vi "dfd_Validate Subband Counts.vi"(8 "error in (no error)":errorcluster, 10 "band counts":i32) -> (0 "error out":errorcluster, 2 "dup band counts":i32)   [LabVIEW 2017, in "NI_DigFilter_FilterBank.lvlib"]
uses:
  <vilib>/addons/Digital Filter Design/NI_DigFilter_FilterBank.lvlib
  <vilib>/addons/Digital Filter Design/_Misc.llb/dfd_Error Handlers (Single).vi
  <vilib>/addons/Digital Filter Design/NI_DigFilterLicensed.lvlib
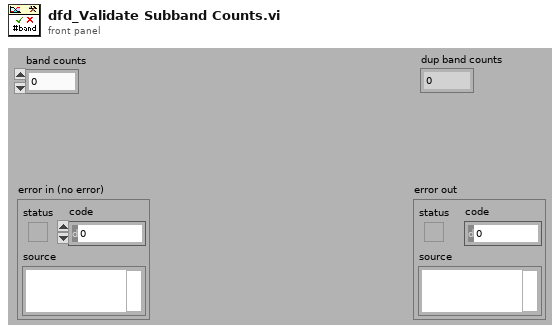
[diagram p1: front panel]
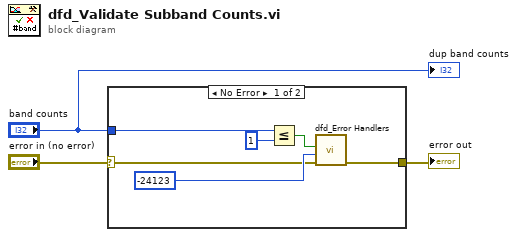
[diagram p0: block diagram]
diagram:
  n1 = case shown="No Error" "error in (no error)" {
    selector: "error in (no error)" -> [w4 w10]
    tunnel: "band counts" -> [w7 _]
    tunnel: [w5 w10] -> w3
    frame No Error {
      n2 = Less Or Equal?(x=w7, y=1) -> (x <= y?=w6:bool)
      n3 = call-poly <vilib>:"dfd_Error Handlers.vi"("error in (no error)"=w4, "error code"=-24123 ("ERR_INVALID_BAND_NUM"), "condition failed?"=w6) -> ("error out"=w5:errorcluster)  [unwired: 8 out]
    }
    frame Error {
    }
  }
  "error out" <- w3
  "dup band counts" <- "band counts"
